vi "Read Binary Config.vi"(4 "Class Name is Included":bool, 6 "byte order (0:big-endian, network order)":T1(ring), 8 "error in (no error)":errorcluster, 10 "Binary":string, 11 "AbsFunc_Two Term_DBL in":refnum<class "AbsFunc_Two Term_DBL.lvclass">) -> (0 "error out":errorcluster, 2 "Remaining":string, 3 "AbsFunc_Two Term_DBL out":refnum<class "AbsFunc_Two Term_DBL.lvclass">)   [LabVIEW 2021, in "AbsFunc_Two Term_DBL.lvclass"]
uses:
  AbsFunc_Two Term_DBL.lvclass
  AbsFunc_Two Term_DBL.lvclass/AbsFunc_Two Term_DBL.ctl
  Abs_Types/Numeric/Abs_Numeric.lvclass
  C:/Program Files (x86)/National Instruments/LabVIEW 2021/vi.lib/TSA/Abstract Data Classes/Abs_Types/Type/Abs_Type.lvclass
  Abs_Types/Double Float/Abs_Double Float.lvclass
  Abs_Types/Type/Abs_Type.lvclass
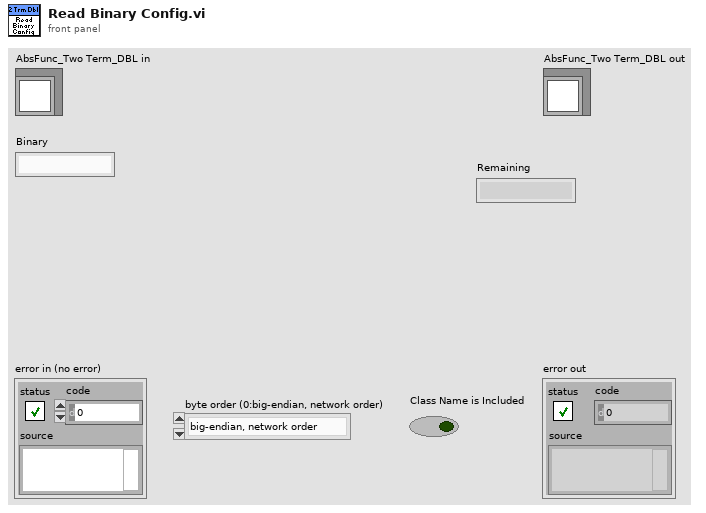
[diagram p1: front panel]
types:
  T1 = enum16{"big-endian, network order", "native, host order", "little-endian"}
  T2 = typedef "AbsFunc_Two Term_DBL.lvclass/Abstract Type.ctl" = refnum<class "Abs_Double Float.lvclass">
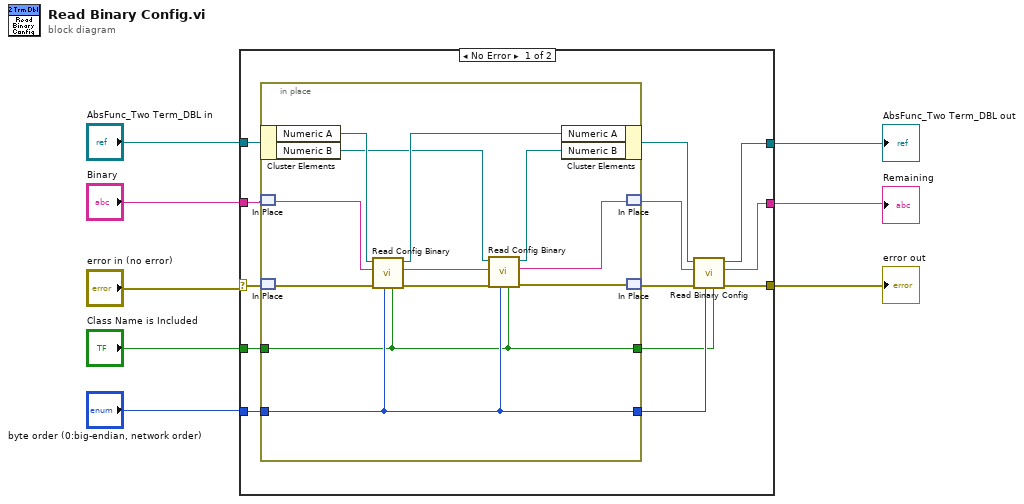
[diagram p0: block diagram]
diagram:
  n1 = case shown="No Error" "error in (no error)" {
    selector: "error in (no error)" -> [w20 w34]
    tunnel: "Binary" -> [w21 w35]
    tunnel: "AbsFunc_Two Term_DBL in" -> [w19 w36]
    tunnel: [w15 w34] -> w1
    tunnel: [w14 w36] -> w3
    tunnel: "Class Name is Included" -> [w13 _]
    tunnel: "byte order (0:big-endian, network order)" -> [w12 _]
    tunnel: [w9 w35] -> w2
    frame No Error {
      n2 = in-place {
        in-place-border: w13 -> [w25]
        in-place-border: w12 -> [w26]
        in-place-border: [w26] -> w11
        in-place-border: [w25] -> w10
        n3 = in-place-cluster #1(w19) -> ("Numeric A"=w32:T2, "Numeric B"=w29:refnum<class "Abs_Numeric.lvclass">)
        n4 = in-place-match #2(w21) -> (w24:string)
        n5 = in-place-match #3(w20) -> (w33:errorcluster)
        n6 = call "Read Config Binary.vi"("Class Name is Included"=w25, "byte order (0:big-endian, network order)"=w26, "error in (no error)"=w33, "Binary"=w24, "Abs_Type in"=w32) -> ("error out"=w30:errorcluster, "Remaining"=w23:string, "Abs_Type out"=w31:T2)  [unwired: 4 in]
        n7 = call "Read Config Binary.vi"("Class Name is Included"=w25, "byte order (0:big-endian, network order)"=w26, "error in (no error)"=w30, "Binary"=w23, "Abs_Type in"=w29) -> ("error out"=w27:errorcluster, "Remaining"=w22:string, "Abs_Type out"=w28:refnum<class "Abs_Numeric.lvclass">)  [unwired: 4 in]
        n8 = in-place-cluster #1("Numeric A"=w31, "Numeric B"=w28) -> (w16:refnum<class "AbsFunc_Two Term_DBL.lvclass">)
        n9 = in-place-match #2(w22) -> (w17:string)
        n10 = in-place-match #3(w27) -> (w18:errorcluster)
      }
      n11 = call-parent "Read Binary Config.vi"("Class Name is Included"=w10, "byte order (0:big-endian, network order)"=w11, "error in (no error)"=w18, "Binary"=w17, "Abs_Type in"=w16) -> ("error out"=w15:errorcluster, "Remaining"=w9:string, "Abs_Type out"=w14:refnum<class "AbsFunc_Two Term_DBL.lvclass">)  [unwired: 4 in]
    }
    frame Error {
    }
  }
  "error out" <- w1
  "AbsFunc_Two Term_DBL out" <- w3
  "Remaining" <- w2
